vi "Population Create.vi"(8 "error in (no error)":errorcluster, 11 "TSP Class in":refnum<class "TSP Class.lvclass">) -> (0 "error out":errorcluster, 3 "TSP Class out":refnum<class "TSP Class.lvclass">)   [LabVIEW 2015, in "TSP Library.lvlib" / "TSP Class.lvclass"]
uses:
  TSP Class.lvclass
  TypeDef/Path.ctl
  TSP Class.lvclass/TSP Class.ctl
  TSP Library.lvlib
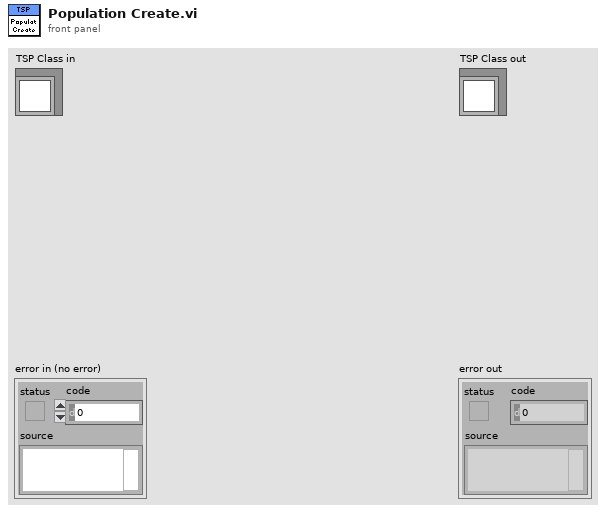
[diagram p1: front panel]
types:
  T1 = typedef "TSP Library.lvlib/Path.ctl" = cluster{"Distance":dbl, "Tour":u16[]}
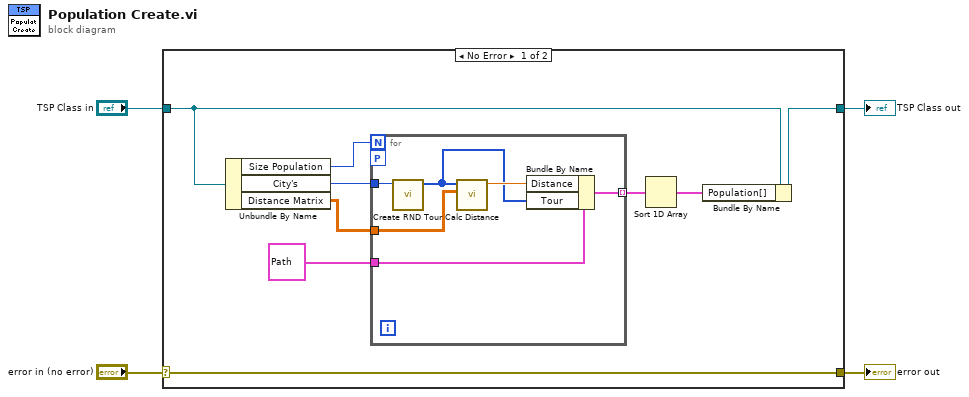
[diagram p0: block diagram]
diagram:
  n1 = case shown="No Error" "error in (no error)" {
    selector: "error in (no error)" -> [w13 w21]
    tunnel: [w13 w21] -> w3
    tunnel: [w8 w20] -> w1
    tunnel: "TSP Class in" -> [w12 w20]
    frame No Error {
      n2 = Unbundle By Name(w12) -> ("Size Population"=w11:u16, "City's"=w6:u16, "Distance Matrix"=w5:dbl[][])
      n3 = for {
        N: w11 -> [_]
        tunnel: w6 -> [w19]
        tunnel: T1 {"Distance"=0.0, "Tour"=[68, 82, 14, 66, 38, 76, 91, 89, 87, 84, 25, 25, 88]} ("Path") -> [w18]
        tunnel: [w15] -> w9 mode=indexing
        workers-P: _ -> [_]
        tunnel: w5 -> [w14]
        n4 = call "Create RND Tour.vi"("City's"=w19) -> ("Tour"=w16:u16[])  [unwired: 10 in]
        n5 = call "Calc Distance.vi"("Distance Matrix"=w14, "Tour"=w16) -> ("Distance"=w17:dbl)  [unwired: 9 in]
        n6 = Bundle By Name(cluster=w18, "Distance"=w17, "Tour"=w16) -> (w15:T1)
      }
      n7 = Sort 1D Array(array=w9) -> (sorted array=w7:T1[])
      n8 = Bundle By Name(cluster=w12, "Population[]"=w7) -> (w8:refnum<class "TSP Class.lvclass">)
    }
    frame Error {
    }
  }
  "error out" <- w3
  "TSP Class out" <- w1
